vi "Connect.vi"(8 "error in (no error)":errorcluster, 11 "Gantry 2":refnum<k24>) -> (0 "error out":errorcluster, 3 "Gantry 3":refnum<k24>)   [LabVIEW 2020, in "A3200.lvclass"]
uses:
  A3200.lvclass
  Drivers/Aerotech A3200/Aerotech.lvlib
  C:/Program Files (x86)/Aerotech/A3200/LabVIEW/2010/Bin/Aerotech.A3200.dll
  Program Files (x86)/Aerotech/A3200/LabVIEW/2010/Bin/Aerotech.A3200.dll
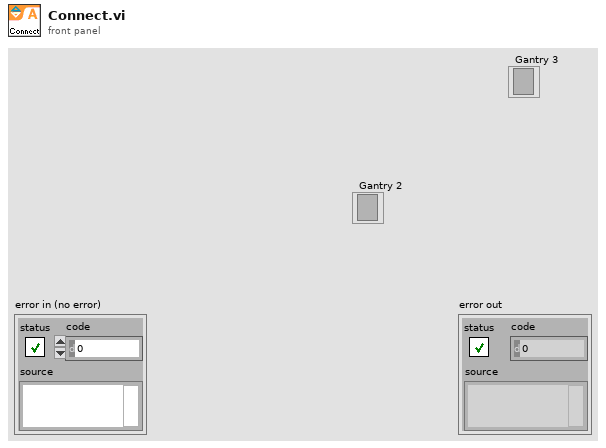
[diagram p1: front panel]
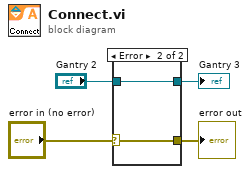
[diagram p0: block diagram]
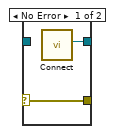
[diagram p2: hidden frame]
diagram:
  n1 = case shown="Error" "error in (no error)" {
    selector: "error in (no error)" -> [w6 w8]
    tunnel: [w6 w8] -> w3
    tunnel: [w5 w7] -> w2
    tunnel: "Gantry 2" -> [_ w7]
    frame No Error {
      n2 = call "Connect.vi"() -> ("controller"=w5:refnum<k24>)  [unwired: 10 in, 1 out]
    }
    frame Error {
    }
  }
  "error out" <- w3
  "Gantry 3" <- w2
